vi "Get ClusterData From LabVIEW Object.vi"(1 "LabVIEW Object":refnum<class>) -> (0 "Flattened Cluster Data":string[](array[string]))   [LabVIEW 2017, in "Composition.lvlib"]
doc: "Returns the private data clusters for each object in the class hierarchy in ascending order (oldest ancestor first)."
uses:
  Composition.lvlib
  <vilib>/Utility/LVClass/Qualified Name Array To Single String.vi
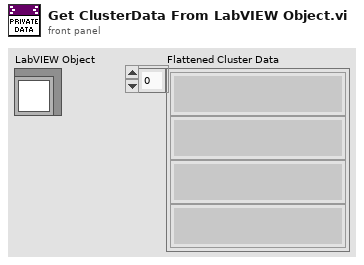
[diagram p1: front panel]
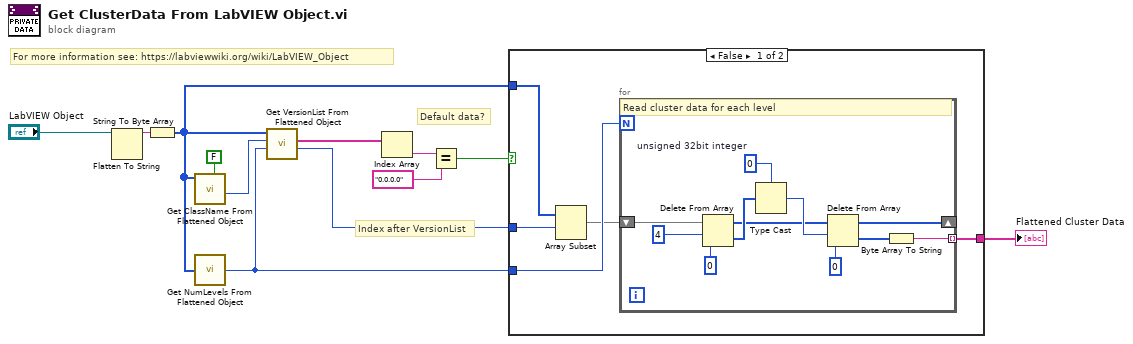
[diagram p0: block diagram]
diagram:
  # "For more information see: https://labviewwiki.org/wiki/LabVIEW_Object"
  # "Index after VersionList"
  # "Default data?"
  n1 = Flatten To String(anything="LabVIEW Object") -> (data string=w6:string)  [unwired: 3 in, 2 out]
  n2 = String To Byte Array(string=w6) -> (unsigned byte array=w2:u8[])
  n3 = call "Get ClassName From Flattened Object.vi"("Read String (T)"=FALSE, "Flattened Object Data"=w2) -> ("Index After ClassName"=w7:i32)  [unwired: 8 in, 1 out]
  n4 = call "Get NumLevels From Flattened Object.vi"("Flattened Object Data"=w2) -> ("Number of Levels"=w5:u32)
  n5 = call "Get VersionList From Flattened Object.vi"("Number of Levels"=w5, "Index After ClassName"=w7, "Flattened Object Data"=w2) -> ("Index After VersionList"=w8:u32, "Version List"=w12:string[])  [unwired: 7 in]
  n6 = Index Array(array=w12) -> (element=w11:string)  [unwired: 1 in]
  n7 = Equal?(x=w11, y="0.0.0.0") -> (x = y?=w9:bool)
  n8 = case shown="False" w9 {
    tunnel: w2 -> [w17 _]
    tunnel: w8 -> [w16 _]
    tunnel: w5 -> [w15 _]
    tunnel: [w14 _] -> w4
    frame False {
      n9 = Array Subset(array=w17, index=w16) -> (w13:u8[])  [unwired: 1 in]
      n10 = for {
        N: w15 -> [_]
        shift-right: [w23] -> _
        shift-left: w13 -> [w27]
        tunnel: [w22] -> w14 mode=indexing
        w26 = u32 0  # unsigned 32bit integer
        # "Read cluster data for each level"
        n11 = Delete From Array(array=w27, length=4, index=0) -> (deleted portion=w25:u8[], array with subset deleted=w19:u8[])
        n12 = Type Cast(type=w26, x=w25) -> (*(type *) &x=w24:u32)
        n13 = Delete From Array(array=w19, length=w24, index=0) -> (deleted portion=w18:u8[], array with subset deleted=w23:u8[])
        n14 = Byte Array To String(unsigned byte array=w18) -> (string=w22:string)
      }
    }
    frame True {
    }
  }
  "Flattened Cluster Data" <- w4
